vi "Execute.vi"(8 "error in":errorcluster, 10 "Shifted Error in":refnum<class "Error.lvclass">, 11 "Error in":refnum<class "Error.lvclass">) -> (0 "error out":errorcluster, 1 "STOP?":bool, 2 "Shifted Error out":refnum<class "Error.lvclass">, 3 "Error out":refnum<class "Error.lvclass">)   [LabVIEW 2019, in "TSC Error.lvlib" / "Error.lvclass"]
doc: "This VI is the template and required override for all Error messages.\n\nInputs:\n-Error in [obj] - the dynamic dispatch input class\n-Shifted Error in [obj] - the shifted error class with shared information\n-error in\n\nOutputs:\n-Error out [obj] - the dynamic dispatch output class\n-Shifted Error in [obj] - the shifted error class with shared information\n-STOP? [Boolean] - the output Boolean used to stop the Error Loop\n-error out\n________________________________________________________________________________\n<b>Code Developed By:</b>\nDaniel Coons\nTechnology Service Corporation\n1983 S Liberty Drive\nBloomington, IN 47403\nPhone: 812 558-7100\ndaniel.coons@tsc.com\nwww.tsc.com\n\n<b>Date Created:</b> 11 AUG 2014\n<b>Date Updated:</b>"
uses:
  Error.lvclass
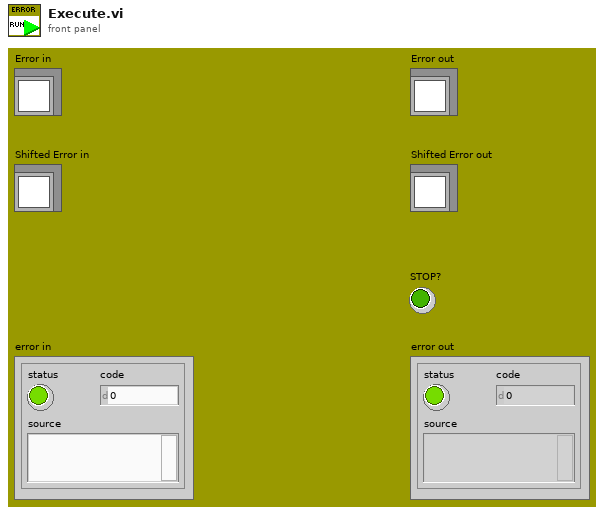
[diagram p1: front panel]
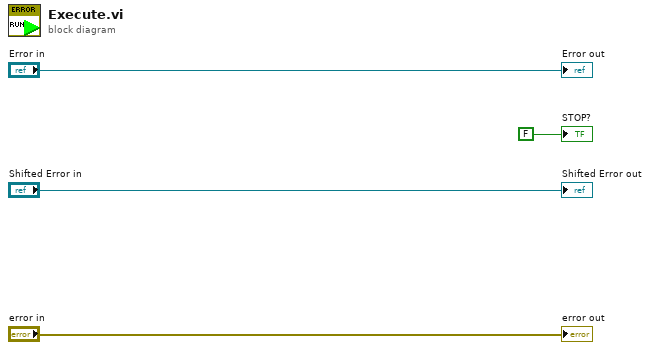
[diagram p0: block diagram]
diagram:
  "Error out" <- "Error in"
  "STOP?" <- FALSE
  "Shifted Error out" <- "Shifted Error in"
  "error out" <- "error in"
